vi "Global.vi"() -> ()   [LabVIEW 2011]
panel:
  in  "PLC":refnum<visa-resource-name>
  in  "SN2_Length":u32
  in  "SN1_Length":u32
  in  "Fix_SN2":T1
  in  "Fix_SN1":T2
  in  "DataBase_Data":T3
  in  "DataBase_Setting":T4
  in  "Scanner2":refnum<visa-resource-name>
  in  "Scanner1":refnum<visa-resource-name>
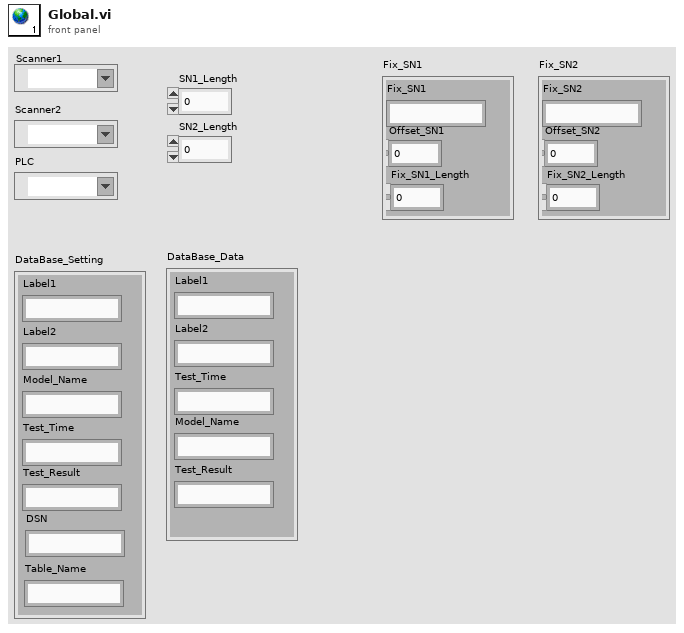
[diagram p1: front panel]
types:
  T1 = cluster{"Fix_SN2":string, "Offset_SN2":u32, "Fix_SN2_Length":u32}
  T2 = cluster{"Fix_SN1":string, "Offset_SN1":u32, "Fix_SN1_Length":u32}
  T3 = cluster{"Label1":string, "Label2":string, "Test_Time":string, "Model_Name":string, "Test_Result":string}
  T4 = cluster{"Label1":string, "Label2":string, "Model_Name":string, "Test_Time":string, "Test_Result":string, "DSN":string, "Table_Name":string}
diagram:
